vi "Set XY Graph Plot Colors.vi"(8 "error in (no error)":errorcluster, 9 "Colors []":u32[](array[colorbox]), 10 "Multiple XY-data in":cluster{"X-array":dbl[], "Y-array":dbl[]}[](array[cluster]) {"Y-array" format="%.2p"; "X-array" format="%.2p"}, 11 "graph_utilities in":refnum<class "graph_utilities.lvclass">) -> (0 "error out":errorcluster, 2 "Multiple XY-data out":cluster{"X-array":dbl[], "Y-array":dbl[]}[](array[cluster]), 3 "graph_utilities out":refnum<class "graph_utilities.lvclass">)   [LabVIEW 2016, in "graph_utilities.lvclass"]
uses:
  graph_utilities.lvclass
  graph_utilities.lvclass/graph_utilities.ctl
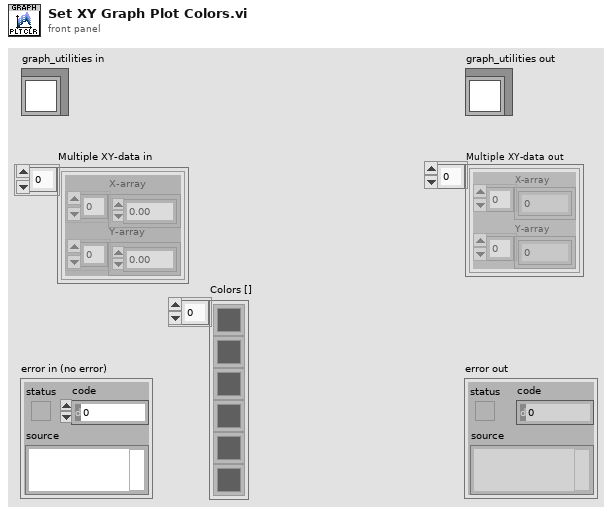
[diagram p1: front panel]
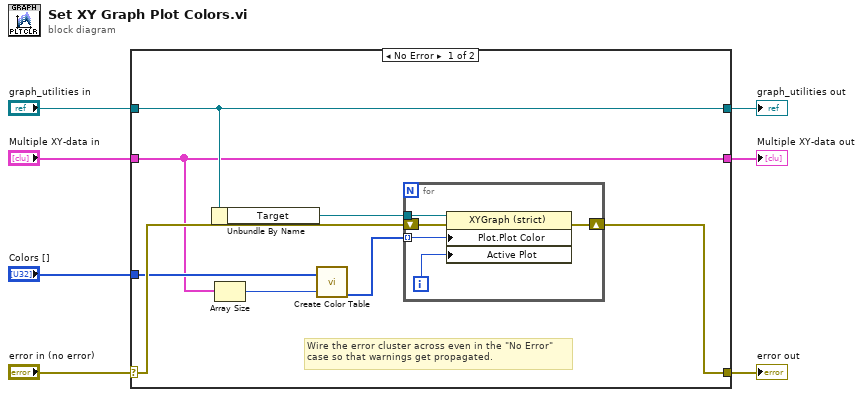
[diagram p0: block diagram]
diagram:
  n1 = case shown="No Error" "error in (no error)" {
    selector: "error in (no error)" -> [w14 w23]
    tunnel: [w13 w23] -> w6
    tunnel: [w15 w22] -> w4
    tunnel: "graph_utilities in" -> [w15 w22]
    tunnel: [w9 w21] -> w2
    tunnel: "Multiple XY-data in" -> [w9 w21]
    tunnel: "Colors []" -> [w11 _]
    frame No Error {
      # "Wire the error cluster across even in the \"No Error\"\ncase so that warnings get propagated."
      n2 = Unbundle By Name(w15) -> ("Target"=w12:refnum<vi>)
      n3 = Array Size(array=w9) -> (size(s)=w8:i32)
      n4 = call "Create Color Table.vi"("Colors []"=w11, "Size"=w8) -> ("Color Tbl"=w10:u32[])  [unwired: 3 out]
      n5 = for {
        tunnel: w12 -> [w18]
        shift-right: [w19] -> w13
        shift-left: w14 -> [w20]
        tunnel: w10 -> [w16] mode=indexing
        i -> [w17]
        n6 = property on="Property Node" class="XYGraph (strict)"(reference=w18, error in=w20, "Plot.Plot Color"=w16, "Active Plot"=w17) -> (error out=w19:errorcluster)  [unwired: 1 out]
      }
    }
    frame Error {
    }
  }
  "error out" <- w6
  "graph_utilities out" <- w4
  "Multiple XY-data out" <- w2
